vi "数据库连接测试.vi"   [LabVIEW 2016]
uses:
  sqlerver.lvclass
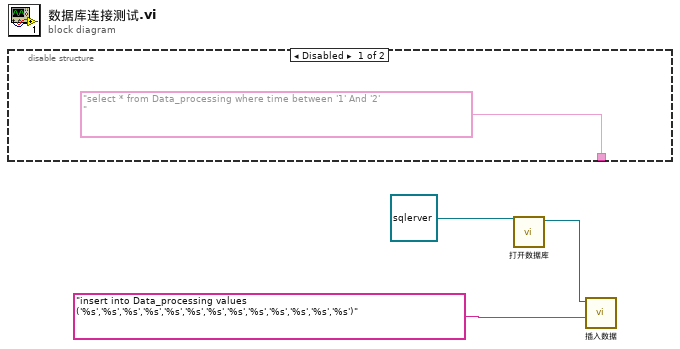
[diagram p0: block diagram]
diagram:
  n1 = disable-structure shown="Disabled" {
    disable-tunnel: ["select * from Data_processing where time between '1' And '2'                                                                " ("格式字符串") _] -> _
    frame Disabled {
    }
    frame Enabled {
    }
  }
  n2 = call-dynamic "打开数据库.vi"("sqlerver in"=refnum<class "sqlerver.lvclass"> refnum ("sqlerver.lvclass")) -> ("sqlerver out"=w2:refnum<class "sqlerver.lvclass">)  [unwired: 9 in, 1 out]
  n3 = call-dynamic "插入数据.vi"("SQL query"="insert into Data_processing values ('%s','%s','%s','%s','%s','%s','%s','%s','%s','%s','%s','%s','%s')" ("格式字符串"), "sqlerver in"=w2) -> ()  [unwired: 8 in, 2 out]
